vi "PZT Set Position-不回调.vi"(8 "Set Position （°/mm）":dbl, 9 "Origin":dbl=5.0, 10 "Range":dbl=10.92, 11 "VISA resource name":refnum<visa-resource-name> caption="VISA资源名称") -> (2 "Current Position （mm  /  °）":dbl, 3 "VISA资源名称输出":refnum<visa-resource-name>)   [LabVIEW 2019]
panel:
  out "Set Position-Real （°/mm）":dbl
  out "初始运动方向":bool
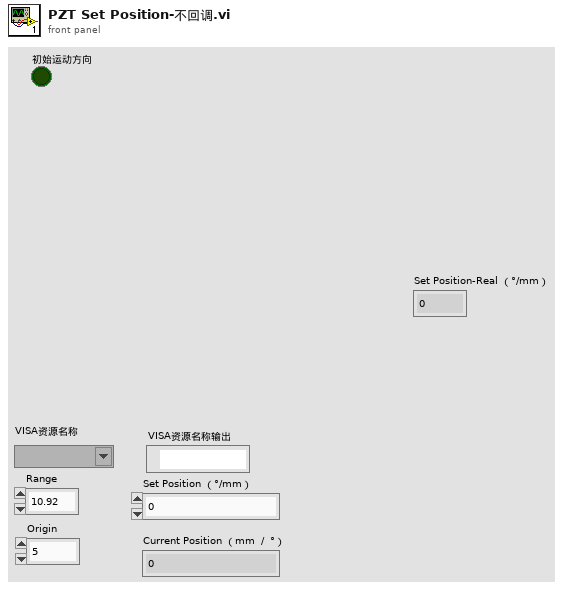
[diagram p1: front panel]
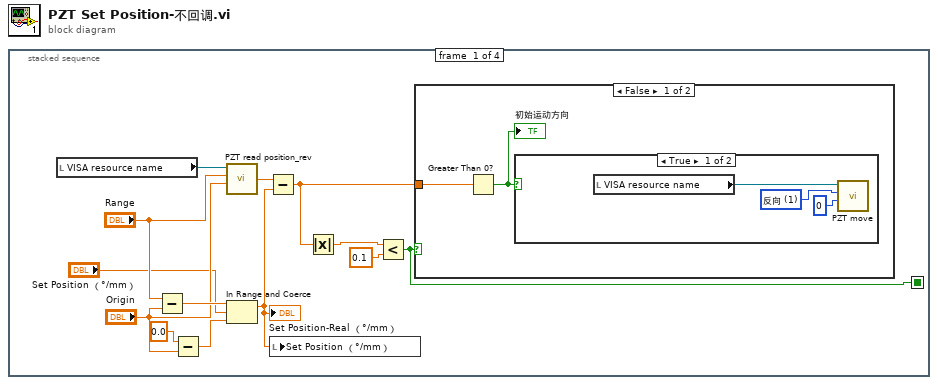
[diagram p0: block diagram]
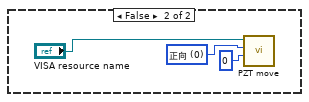
[diagram p2: hidden frame]
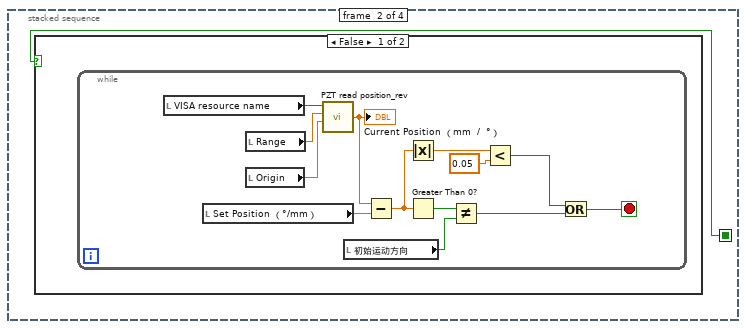
[diagram p4: hidden frame]
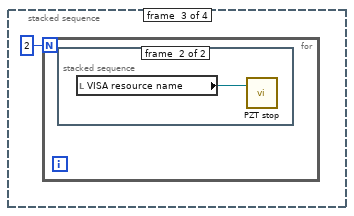
[diagram p6: hidden frame]
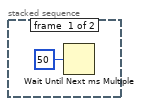
[diagram p7: hidden frame]
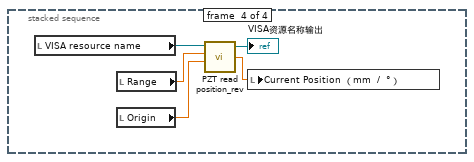
[diagram p8: hidden frame]
diagram:
  n1 = stacked-sequence {
    seq-local: [w9 _ _ _] -> [_ w22 _ _]
    frame #0 {
      n2 = local read "VISA resource name"() -> (w13:refnum<visa-resource-name>)
      n3 = Subtract(x="Range", y="Origin") -> (x-y=w6:dbl)
      n4 = Subtract(x=0.0, y="Origin") -> (x-y=w7:dbl)
      n5 = call "PZT read position_rev.vi"("Origin"="Origin", "Range"="Range", "VISA resource name"=w13) -> ("Current Position （mm  /  °）"=w12:dbl)  [unwired: 1 in, 2 out]
      n6 = In Range and Coerce(upper limit=w6, x="Set Position （°/mm）", lower limit=w7) -> (coerced(x)=w1:dbl)  [unwired: 1 out]
      "Set Position-Real （°/mm）" <- w1
      n7 = Subtract(x=w12, y=w1) -> (x-y=w10:dbl)
      n8 = local write "Set Position （°/mm）"(w1) -> ()
      n9 = Absolute Value(x=w10) -> (abs(x)=w8:dbl)
      n10 = Less?(x=w8, y=0.1) -> (x < y?=w9:bool)
      n11 = case shown="False" w9 {
        tunnel: w10 -> [w14 _]
        frame False {
          n12 = Greater Than 0?(x=w14) -> (x > 0?=w15:bool)
          "初始运动方向" <- w15
          n13 = case shown="True" w15 {
            frame True {
              w18 = u16 1 items=["正向", "反向"] ("移动方向")
              n14 = local read "VISA resource name"() -> (w16:refnum<visa-resource-name>)
              n15 = call "PZT move.vi"("移动步数"=0, "移动方向"=w18, "VISA resource name"=w16) -> ()  [unwired: 1 in, 2 out]
            }
            frame False {
              w20 = u16 0 items=["正向", "反向"] ("移动方向")
              n16 = call "PZT move.vi"("移动步数"=0, "移动方向"=w20, "VISA resource name"="VISA resource name") -> ()  [unwired: 1 in, 2 out]
            }
          }
        }
        frame True {
        }
      }
    }
    frame #1 {
      n17 = case shown="False" w22 {
        frame False {
          n18 = while {
            stop <- w25 stop-if-true
            n19 = local read "VISA resource name"() -> (w35:refnum<visa-resource-name>)
            n20 = local read "Set Position （°/mm）"() -> (w31:dbl)
            n21 = local read "Range"() -> (w34:dbl)
            n22 = local read "Origin"() -> (w33:dbl)
            n23 = call "PZT read position_rev.vi"("Origin"=w33, "Range"=w34, "VISA resource name"=w35) -> ("Current Position （mm  /  °）"=w32:dbl)  [unwired: 1 in, 2 out]
            "Current Position （mm  /  °）" <- w32
            n24 = local read "初始运动方向"() -> (w28:bool)
            n25 = Subtract(x=w32, y=w31) -> (x-y=w27:dbl)
            n26 = Absolute Value(x=w27) -> (abs(x)=w30:dbl)
            n27 = Greater Than 0?(x=w27) -> (x > 0?=w26:bool)
            n28 = Not Equal?(x=w26, y=w28) -> (x != y?=w23:bool)
            n29 = Less?(x=w30, y=0.05) -> (x < y?=w24:bool)
            n30 = Or(x=w24, y=w23) -> (x .or. y?=w25:bool)
          }
        }
        frame True {
        }
      }
    }
    frame #2 {
      n31 = for {
        N: 2 -> [_]
        n32 = stacked-sequence {
          frame #0 {
            n33 = Wait Until Next ms Multiple(millisecond multiple=u32 50 ("毫秒倍数")) -> ()  [unwired: 1 out]
          }
          frame #1 {
            n34 = local read "VISA resource name"() -> (w38:refnum<visa-resource-name>)
            n35 = call "PZT stop.vi"("VISA resource name"=w38) -> ()  [unwired: 1 in, 2 out]
          }
        }
      }
    }
    frame #3 {
      n36 = local read "VISA resource name"() -> (w43:refnum<visa-resource-name>)
      n37 = local read "Range"() -> (w42:dbl)
      n38 = local read "Origin"() -> (w41:dbl)
      n39 = call "PZT read position_rev.vi"("Origin"=w41, "Range"=w42, "VISA resource name"=w43) -> ("Current Position （mm  /  °）"=w40:dbl, "VISA资源名称输出"=→"VISA资源名称输出":refnum<visa-resource-name>)  [unwired: 1 in, 1 out]
      n40 = local write "Current Position （mm  /  °）"(w40) -> ()
    }
  }
